vi "Digital input.vi"(8 "error in":errorcluster, 11 "DAQmx InPut Setting":T1) -> (0 "error out":errorcluster, 1 "Exit":bool)   [LabVIEW 2015]
uses:
  <vilib>/DAQmx/read.llb/DAQmx Read (Digital 1D Bool 1Chan 1Samp).vi
  <vilib>/DAQmx/create/channels.llb/DAQmx Create Channel (DI-Digital Input).vi
  Galobal variable_TI.vi
  <vilib>/DAQmx/miscellaneous.llb/DAQmx Fill In Error Info.vi
panel:
  out "output array":bool[](array[boolean])
  out "error out 2":errorcluster
  out "status":bool
  out "Array":bool[](array[boolean])
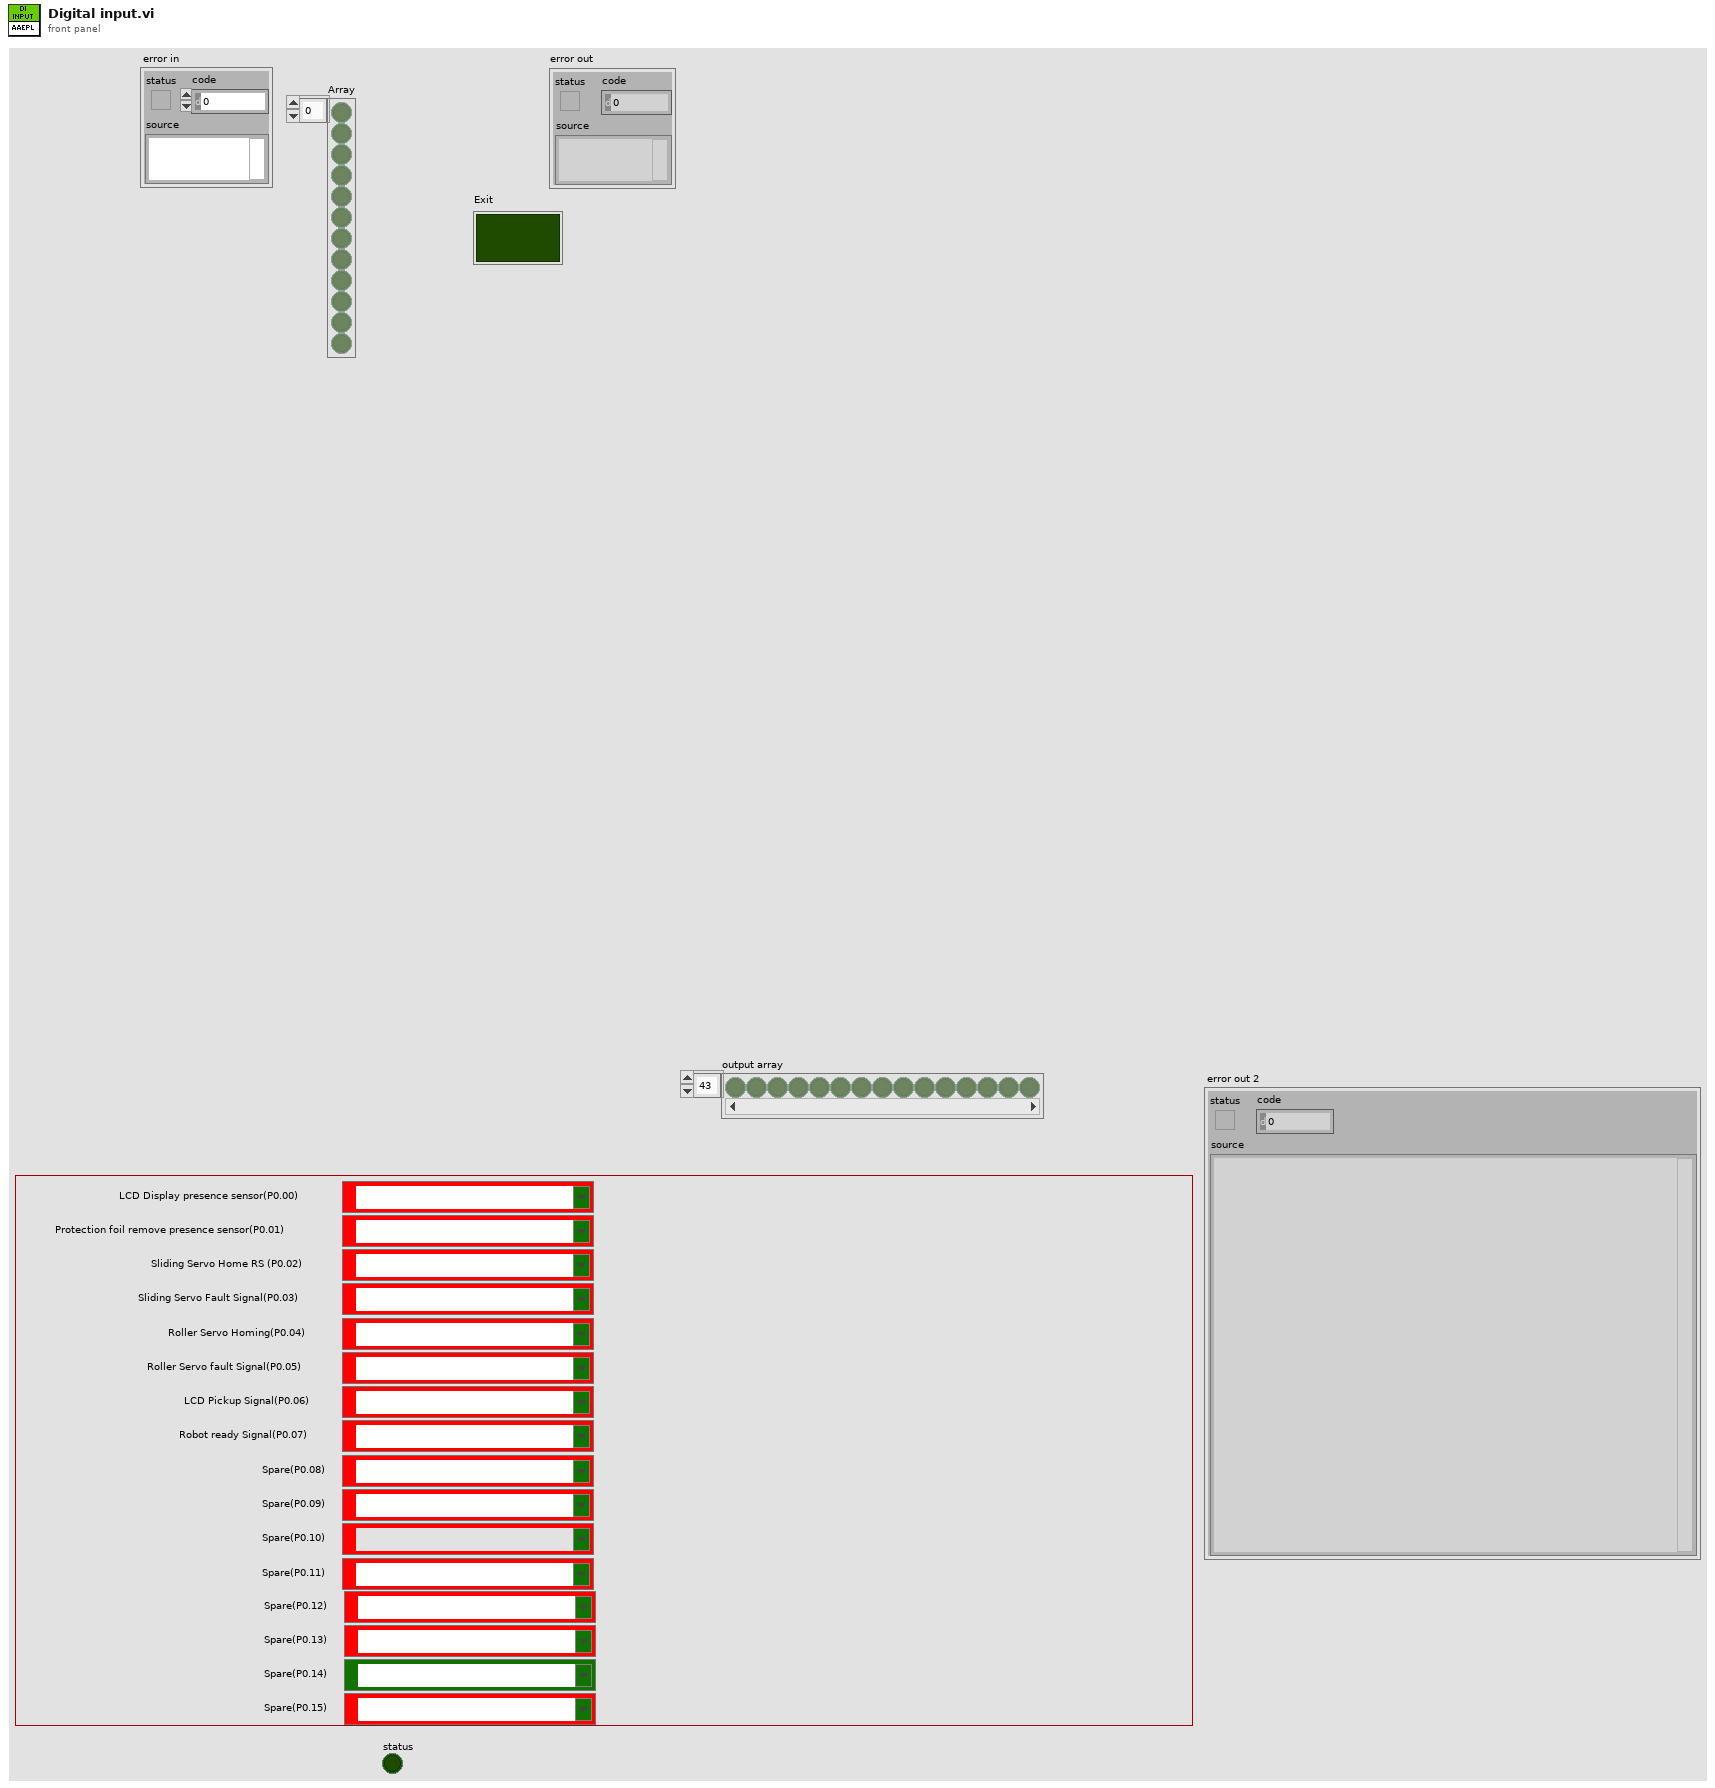
[diagram p1: front panel]
types:
  T1 = cluster{"DAQmx InPut_00":tag, "DAQmx InPut_01":tag, "DAQmx InPut_02":tag, "DAQmx InPut_03":tag, "DAQmx InPut_04":tag, "DAQmx InPut_05":tag, "DAQmx InPut_06":tag, "DAQmx InPut_07":tag, "DAQmx InPut_08":tag, "DAQmx InPut_09":tag, "DAQmx InPut_10":tag, "DAQmx InPut_11":tag, "DAQmx InPut_12":tag, "DAQmx InPut_13":tag, "DAQmx InPut_14":tag, "DAQmx InPut_15":tag}
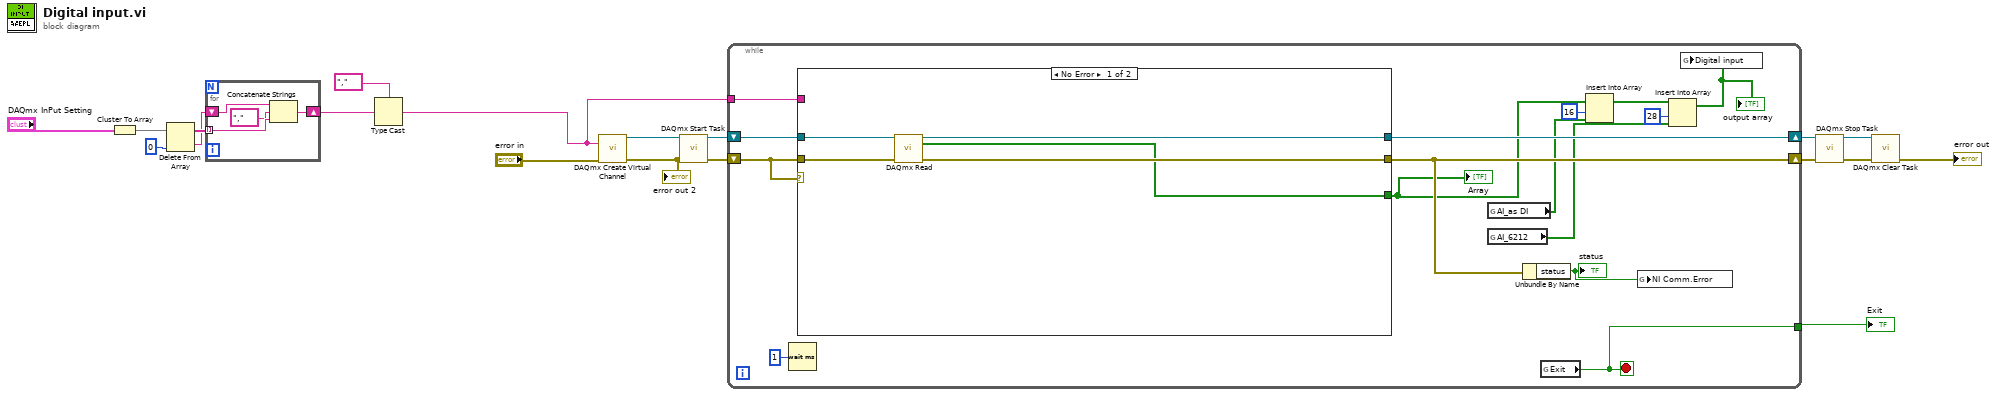
[diagram p0: block diagram]
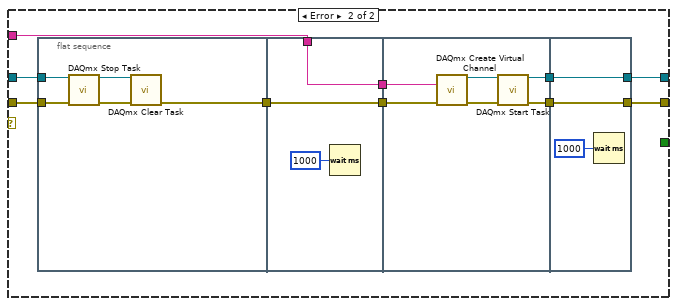
[diagram p2: hidden frame]
diagram:
  n1 = Cluster To Array(cluster="DAQmx InPut Setting") -> (array=w9:tag[])
  n2 = Delete From Array(array=w9, index=0) -> (deleted portion=w6:tag, array with subset deleted=w8:tag[])  [unwired: 1 in]
  n3 = for {
    tunnel: w8 -> [w22] mode=indexing
    shift-right: [w20] -> w4
    shift-left: w6 -> [w23]
    n4 = Concatenate Strings(w23, tag "," ("1."), w22) -> (w20:string)
  }
  n5 = Type Cast(type=tag "," ("1."), x=w4) -> (*(type *) &x=w3:tag)
  n6 = call-poly <vilib>:"DAQmx Create Virtual Channel.vi"("lines"=w3, "error in"="error in") -> ("task out"=w19:refnum<k21>, "error out"=w18:errorcluster)  [unwired: 3 in, 9 out]
  "error out 2" <- w18
  n7 = call <vilib>:"DAQmx Start Task.vi"("task/channels in"=w19, "error in"=w18) -> ("task out"=w16:refnum<k21>, "error out"=w17:errorcluster)  [unwired: 12 out]
  n8 = while {
    shift-right: [w33] -> w13
    shift-left: w17 -> [w38]
    shift-right: [w36] -> w12
    shift-left: w16 -> [w37]
    tunnel: w3 -> [w35]
    tunnel: [w34] -> w10
    stop <- w34 stop-if-true
    n9 = Wait (ms)(milliseconds to wait=u32 1) -> ()  [unwired: 1 out]
    n10 = case shown="No Error" w38 {
      tunnel: w38 -> [w43 w52]
      tunnel: w37 -> [w42 w53]
      tunnel: [w41 w45] -> w33
      tunnel: [w40 w44] -> w36
      tunnel: w35 -> [_ w48]
      tunnel: [w39 _] -> w31
      frame No Error {
        n11 = call-poly <vilib>:"DAQmx Read.vi"("task/channels in"=w42, "error in"=w43) -> ("task out"=w40:refnum<k21>, "data"=w39:bool[], "error out"=w41:errorcluster)  [unwired: 1 in, 10 out]
      }
      frame Error {
        n12 = flat-sequence {
          tunnel: w53 -> [w56]
          tunnel: w52 -> [w55]
          tunnel: [w54] -> w51
          tunnel: w51 -> [w60]
          tunnel: [w60] -> w50
          tunnel: [w59] -> w49
          tunnel: w48 -> [w59]
          tunnel: w50 -> [w65]
          tunnel: w49 -> [w64]
          tunnel: [w63] -> w47
          tunnel: [w62] -> w46
          tunnel: w47 -> [w70]
          tunnel: w46 -> [w69]
          tunnel: [w70] -> w45
          tunnel: [w69] -> w44
          frame #0 {
            n13 = call <vilib>:"DAQmx Stop Task.vi"("task/channels in"=w56, "error in"=w55) -> ("task out"=w57:refnum<k21>, "error out"=w58:errorcluster)  [unwired: 12 in]
            n14 = call <vilib>:"DAQmx Clear Task.vi"("task in"=w57, "error in"=w58) -> ("error out"=w54:errorcluster)  [unwired: 13 in]
          }
          frame #1 {
            n15 = Wait (ms)(milliseconds to wait=u32 1000) -> ()  [unwired: 1 out]
          }
          frame #2 {
            n16 = call-poly <vilib>:"DAQmx Create Virtual Channel.vi"("lines"=w64, "error in"=w65) -> ("task out"=w66:refnum<k21>, "error out"=w67:errorcluster)  [unwired: 3 in, 9 out]
            n17 = call <vilib>:"DAQmx Start Task.vi"("task/channels in"=w66, "error in"=w67) -> ("task out"=w62:refnum<k21>, "error out"=w63:errorcluster)  [unwired: 12 out]
          }
          frame #3 {
            n18 = Wait (ms)(milliseconds to wait=u32 1000) -> ()  [unwired: 1 out]
          }
        }
      }
    }
    "Array" <- w31
    n19 = global read "Galobal variable_TI.vi" "AI_as DI"() -> (w29:bool[])
    n20 = global read "Galobal variable_TI.vi" "AI_6212"() -> (w26:bool[])
    n21 = Unbundle By Name(w33) -> ("status"=w32:bool)
    "status" <- w32
    n22 = global read "Galobal variable_TI.vi" "Exit"() -> (w34:bool)
    n23 = Insert Into Array(array=w31, index=16, new element=w29) -> (w27:bool[])
    n24 = global write "Galobal variable_TI.vi" "NI Comm.Error"(w32) -> ()
    n25 = Insert Into Array(array=w27, index=28, new element=w26) -> (w25:bool[])
    "output array" <- w25
    n26 = global write "Galobal variable_TI.vi" "Digital input"(w25) -> ()
  }
  "Exit" <- w10
  n27 = call <vilib>:"DAQmx Stop Task.vi"("task/channels in"=w12, "error in"=w13) -> ("task out"=w14:refnum<k21>, "error out"=w15:errorcluster)  [unwired: 12 in]
  n28 = call <vilib>:"DAQmx Clear Task.vi"("task in"=w14, "error in"=w15) -> ("error out"=→"error out":errorcluster)  [unwired: 13 in]
